vi "DSF.Simulation.Custom Device.Shutdown.vi"(8 "error in (no error)":errorcluster, 11 "Simulated VeriStand Custom Device in":refnum<class "Simulated VeriStand Custom Device.lvclass">) -> (0 "error out":errorcluster, 3 "Simulated VeriStand Custom Device out":refnum<class "Simulated VeriStand Custom Device.lvclass">)   [LabVIEW 2016, in "Simulated VeriStand Custom Device.lvclass"]
uses:
  Simulated VeriStand Custom Device.lvclass
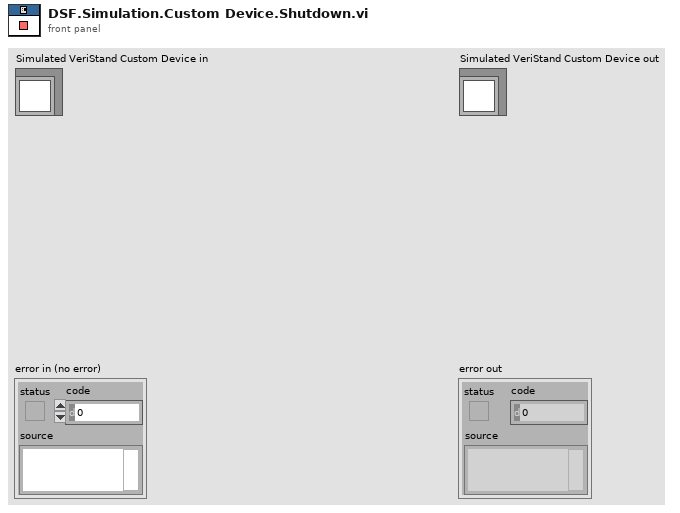
[diagram p1: front panel]
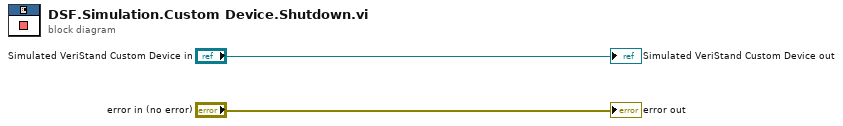
[diagram p0: block diagram]
diagram:
  "error out" <- "error in (no error)"
  "Simulated VeriStand Custom Device out" <- "Simulated VeriStand Custom Device in"
